vi "Process adapted triangles (full).vi"(1 "Triangles in":T1[](array[typedef])) -> (0 "Triangles out":T1[](array[typedef]))   [LabVIEW 2014]
doc: "This VI must be run after any alteration to the triangles geometry involving scaling and rotation.\nThere is no need to run this VI after applying a translation."
uses:
  Typedefs/Triangle.ctl
  Subroutines/Dot product.vi
panel:
  # "PN 29/03/2015"
  # "Vertices"
  # "Edges"
  # "Unit normal"
  # "Edge unit normals"
  # "Vertices"
  # "Edges"
  # "Unit normal"
  # "Edge unit normals"
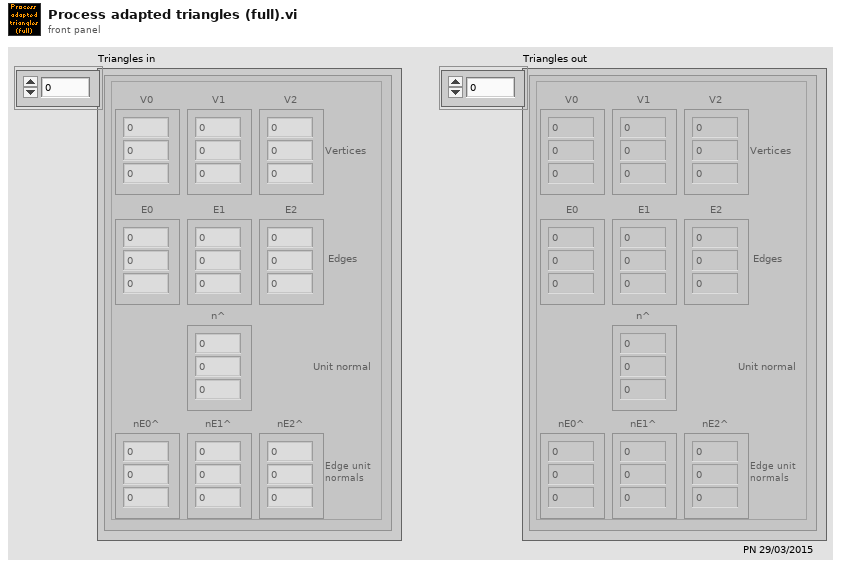
[diagram p1: front panel]
types:
  T1 = typedef "Triangle.ctl" = cluster{"V0":sgl[], "V1":sgl[], "V2":sgl[], "E0":sgl[], "E1":sgl[], "E2":sgl[], "n^":sgl[], "nE0^":sgl[], "nE1^":sgl[], "nE2^":sgl[]}
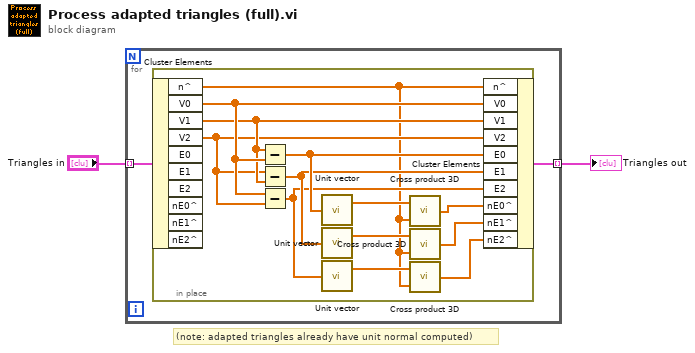
[diagram p0: block diagram]
diagram:
  # "(note: adapted triangles already have unit normal computed)"
  n1 = for {
    tunnel: "Triangles in" -> [w4] mode=indexing
    tunnel: [w3] -> w1 mode=indexing
    n2 = in-place {
      n3 = in-place-cluster #1(w4) -> ("n^"=w5:sgl[], "V0"=w14:sgl[], "V1"=w13:sgl[], "V2"=w12:sgl[])  [unwired: 6 out]
      n4 = Subtract(x=w13, y=w14) -> (x-y=w11:sgl[])
      n5 = Subtract(x=w12, y=w13) -> (x-y=w10:sgl[])
      n6 = Subtract(x=w14, y=w12) -> (x-y=w9:sgl[])
      n7 = call "Unit vector.vi"("Vector"=w11) -> ("Unit vector"=w15:sgl[])  [unwired: 1 out]
      n8 = call "Unit vector.vi"("Vector"=w10) -> ("Unit vector"=w17:sgl[])  [unwired: 1 out]
      n9 = call "Unit vector.vi"("Vector"=w9) -> ("Unit vector"=w16:sgl[])  [unwired: 1 out]
      n10 = call "Cross product 3D.vi"("B"=w5, "A"=w15) -> ("A x B"=w8:sgl[])
      n11 = call "Cross product 3D.vi"("B"=w5, "A"=w17) -> ("A x B"=w7:sgl[])
      n12 = call "Cross product 3D.vi"("B"=w5, "A"=w16) -> ("A x B"=w6:sgl[])
      n13 = in-place-cluster #1("n^"=w5, "V0"=w14, "V1"=w13, "V2"=w12, "E0"=w11, "E1"=w10, "E2"=w9, "nE0^"=w8, "nE1^"=w7, "nE2^"=w6) -> (w3:T1)
    }
  }
  "Triangles out" <- w1
